vi "Event Handler.vi"(8 "error in (no error)":errorcluster, 10 "Stop Event Handler":refnum<user-event>, 11 "ScrollingList in":refnum<class "ScrollingList.lvclass">) -> (0 "error out":errorcluster)   [LabVIEW 2019, in "ScrollingList.lvclass"]
doc: "The <b>Event Handler VI</b> is a dynamic dispatch VI that should be overwritten if events are needed to create the enhanced QControl. \n\nBy inheriting from the main Control.lvclass the overwritten <b>Event Handler VI</b> will be launched asynchronously in the initialization of the QControl.\n<b> </b> <b> </b>\n©2016 Q Software Innovations, LLC (QSI)\nwritten by Quentin Alldredge\nproduced in LabVIEW 2015\n\nsupport@qsoftwareinnovations.com\nwww.qsoftwareinnovations.com\n\nAll rights reserved.\n\nRedistribution and use in source and binary forms, with or without modification, are permitted provided that the following conditions are met:\n\n * Redistributions of source code must retain the above copyright notice, this list of conditions and the following disclaimer.\n * Redistributions in binary form must reproduce the above copyright notice, this list of conditions and the following disclaimer in the documentation and/or other materials provided with the distribution.\n * Neither the name of Q Software Innovations, LLC. nor the names of its contributors may be used to endorse or promote products derived from this software without specific prior written permission.\n\nTHIS SOFTWARE IS PROVIDED BY THE COPYRIGHT HOLDERS AND CONTRIBUTORS \"AS IS\" AND ANY EXPRESS OR IMPLIED WARRANTIES, INCLUDING, BUT NOT LIMITED TO, THE IMPLIED WARRANTIES OF MERCHANTABILITY AND FITNESS FOR A PARTICULAR PURPOSE ARE DISCLAIMED. IN NO EVENT SHALL THE COPYRIGHT OWNER OR CONTRIBUTORS BE LIABLE FOR ANY DIRECT, INDIRECT, INCIDENTAL, SPECIAL, EXEMPLARY, OR CONSEQUENTIAL DAMAGES (INCLUDING, BUT NOT LIMITED TO, PROCUREMENT OF SUBSTITUTE GOODS OR SERVICES; LOSS OF USE, DATA, OR PROFITS; OR BUSINESS INTERRUPTION) HOWEVER CAUSED AND ON ANY THEORY OF LIABILITY, WHETHER IN CONTRACT, STRICT LIABILITY, OR TORT (INCLUDING NEGLIGENCE OR OTHERWISE) ARISING IN ANY WAY OUT OF THE USE OF THIS SOFTWARE, EVEN IF ADVISED OF THE POSSIBILITY OF SUCH DAMAGE."
uses:
  ScrollingList.lvclass
  ScrollingList.lvclass/ScrollingList.ctl
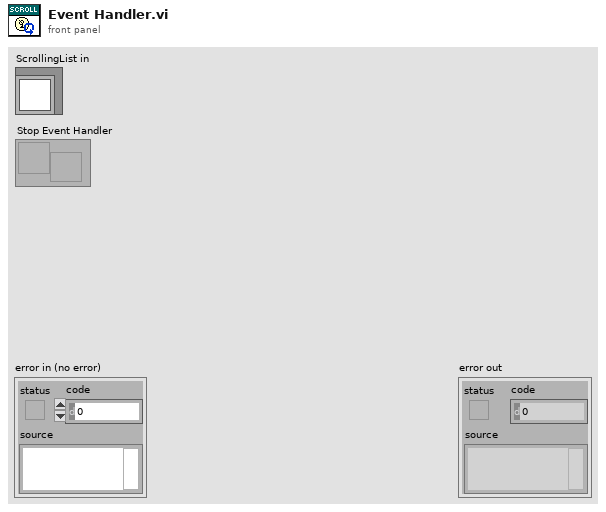
[diagram p1: front panel]
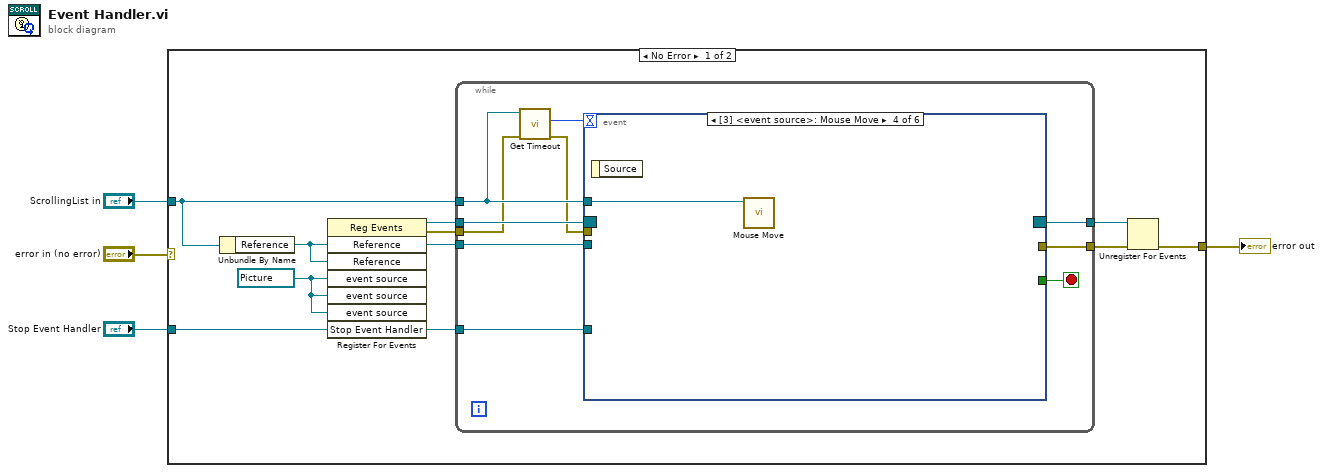
[diagram p0: block diagram]
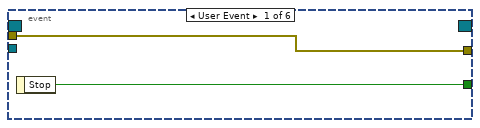
[diagram p2: hidden frame]
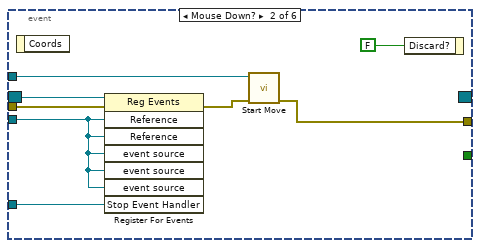
[diagram p3: hidden frame]
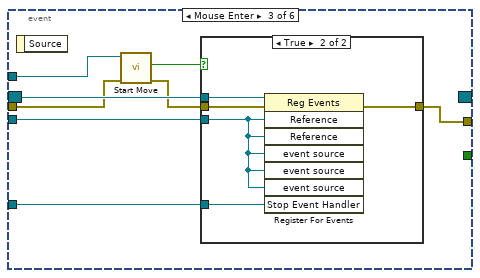
[diagram p4: hidden frame]
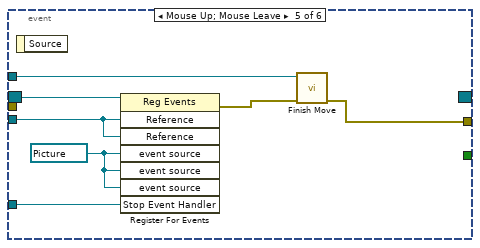
[diagram p6: hidden frame]
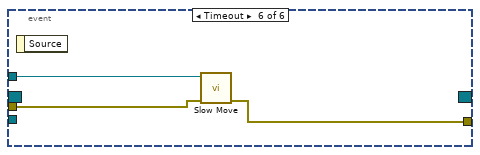
[diagram p7: hidden frame]
diagram:
  n1 = case shown="No Error" "error in (no error)" {
    selector: "error in (no error)" -> [_ w59]
    tunnel: [w10 w59] -> w3
    tunnel: "ScrollingList in" -> [w8 _]
    tunnel: "Stop Event Handler" -> [w6 _]
    frame No Error {
      w7 = refnum<vi> refnum ("event source")
      n2 = Unbundle By Name(w8) -> ("Reference"=w5:refnum<vi>)
      n3 = register-events(w5, w5, w7, w7, w7, w6) -> (reference out=w13:refnum<event-registration>, error out=w12:errorcluster)  [unwired: 2 in]
      n4 = while {
        tunnel: w13 -> [w23]
        tunnel: w12 -> [w14]
        tunnel: [w22] -> w11
        tunnel: [w20] -> w9
        tunnel: w5 -> [w19]
        tunnel: w8 -> [w16]
        tunnel: w6 -> [w18]
        stop <- w21 stop-if-true
        n5 = call "Get Timeout.vi"("error in (no error)"=w14, "ScrollingList in"=w16) -> ("error out"=w15:errorcluster, "Timeout"=w17:i32)  [unwired: 7 in, 1 out]
        n6 = event shown="[3] <event source>: Mouse Move" {
          selector: w23 -> [_ w33 w41 _ w55 _]
          dyn-events: [_ _ _ _ _ _] -> w20
          timeout: w17 -> [_ _ _ _ _ _]
          tunnel: w16 -> [_ w31 w40 w48 w51 w58]
          tunnel: w15 -> [w25 w30 w37 _ _ w57]
          tunnel: [w25 w27 w35 _ w49 w56] -> w22
          tunnel: [w24 _ _ _ _ _] -> w21
          tunnel: w19 -> [_ w28 w38 _ w54 _]
          tunnel: w18 -> [_ w29 w39 _ w52 _]
          event User Event {
            n7 = event-data() -> ("Stop"=w24:bool)  [unwired: 1 in]
          }
          event Mouse Down? {
            n8 = event-data() -> ()  [unwired: 1 in, 1 out]
            n9 = register-events(reference=w33, error in=w30, w28, w28, w28, w28, w28, w29) -> (error out=w26:errorcluster)  [unwired: 1 out]
            n10 = call "Start Move.vi"("error in (no error)"=w26, "ScrollingList in"=w31) -> ("error out"=w27:errorcluster)  [unwired: 7 in, 2 out]
            n11 = event-data("Discard?"=FALSE) -> ()  [unwired: 1 in, 1 out]
          }
          event Mouse Enter {
            n12 = event-data() -> ()  [unwired: 1 in, 1 out]
            n13 = call "Start Move.vi"("error in (no error)"=w37, "ScrollingList in"=w40) -> ("error out"=w36:errorcluster, "Button Down"=w34:bool)  [unwired: 7 in, 1 out]
            n14 = case shown="True" w34 {
              tunnel: w41 -> [_ w47]
              tunnel: w39 -> [_ w46]
              tunnel: w38 -> [_ w45]
              tunnel: w36 -> [w42 w44]
              tunnel: [w42 w43] -> w35
              frame False {
              }
              frame True {
                n15 = register-events(reference=w47, error in=w44, w45, w45, w45, w45, w45, w46) -> (error out=w43:errorcluster)  [unwired: 1 out]
              }
            }
          }
          event Mouse Move {
            n16 = event-data() -> ()  [unwired: 1 in, 1 out]
            n17 = call "Mouse Move.vi"("ScrollingList in"=w48) -> ()  [unwired: 9 in, 2 out]
          }
          event Mouse Up; Mouse Leave {
            w53 = refnum<vi> refnum ("event source")
            n18 = event-data() -> ()  [unwired: 1 in, 1 out]
            n19 = register-events(reference=w55, w54, w54, w53, w53, w53, w52) -> (error out=w50:errorcluster)  [unwired: 1 in, 1 out]
            n20 = call "Finish Move.vi"("error in (no error)"=w50, "ScrollingList in"=w51) -> ("error out"=w49:errorcluster)  [unwired: 8 in, 1 out]
          }
          event Timeout {
            n21 = event-data() -> ()  [unwired: 1 in, 1 out]
            n22 = call "Slow Move.vi"("error in (no error)"=w57, "ScrollingList in"=w58) -> ("error out"=w56:errorcluster)  [unwired: 8 in, 1 out]
          }
        }
      }
      n23 = Unregister For Events(event registration refnum=w9, error in=w11) -> (error out=w10:errorcluster)
    }
    frame Error {
    }
  }
  "error out" <- w3
